vi "DataPacker_ConnectToMIDAS.vi"(8 "error in (no error)":errorcluster, 11 "DataPacker in":refnum<class "DataPacker.lvclass">) -> (0 "error out":errorcluster, 2 "MIDAS Reply":string, 3 "DataPacker out":refnum<class "DataPacker.lvclass">)   [LabVIEW 2018, in "feGEM DataPacker.lvlib" / "DataPacker.lvclass"]
uses:
  DataPacker.lvclass
  DataPacker.lvclass/DataPacker.ctl
  DataStructures/GEM_BANK_ARRAY.lvclass
  DataStructures/GEM_BANK_CLUSTER_typedef.ctl
  DataStructures/GEM_DATA_cluster_typedef.ctl
  5450c936-4932-4056-bb20-e5a86d0e2a98.vi
  feGEM DataPacker.lvlib
panel:
  out "Hostname of this PC":string
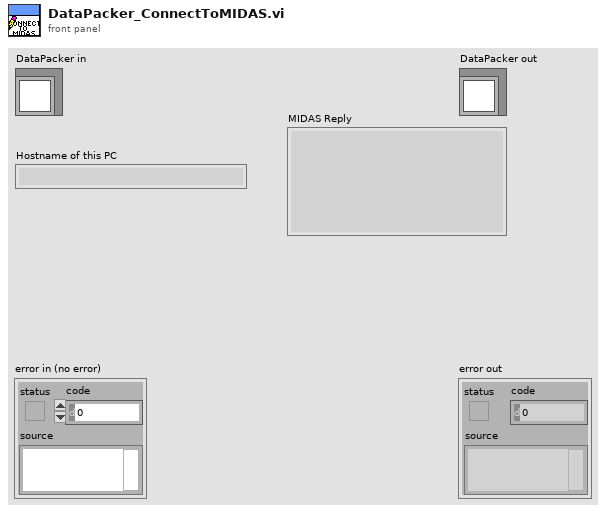
[diagram p1: front panel]
types:
  T1 = typedef "feGEM DataPacker.lvlib/GEM_BANK_CLUSTER_typedef.ctl" = cluster{"Category":string, "Variable Name":string, "Equipment description":string, "History Settings":u16, "Period to update history plots":u16, "GEM_DATA Cluster":T2}
  T2 = typedef "feGEM DataPacker.lvlib/GEM_DATA_cluster_typedef.ctl" = cluster{"DataType":string, "Formatted Data":u8[], "data byte order (Little Endian prefered)":enum16{"big-endian, network order", "native, host order", "little-endian"}}
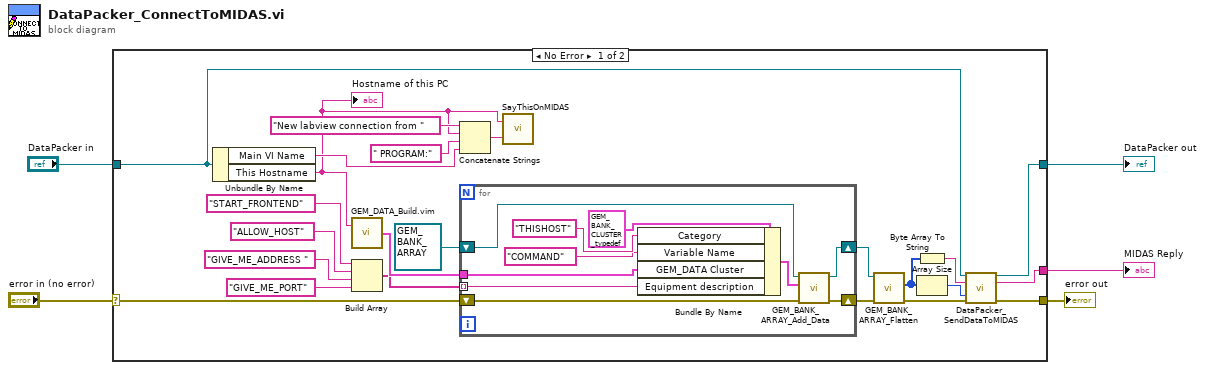
[diagram p0: block diagram]
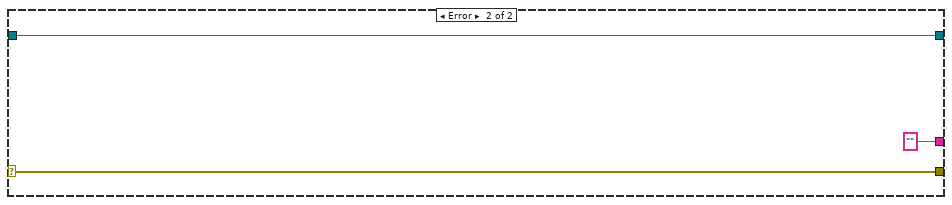
[diagram p2: hidden frame]
diagram:
  n1 = case shown="No Error" "error in (no error)" {
    selector: "error in (no error)" -> [w20 w40]
    tunnel: [w16 w40] -> w4
    tunnel: [w19 w41] -> w2
    tunnel: "DataPacker in" -> [w12 w41]
    tunnel: [w11 "" ("MIDAS Reply")] -> w1
    frame No Error {
      n2 = Unbundle By Name(w12) -> ("Main VI Name"=w10:string, "This Hostname"=w6:string)
      "Hostname of this PC" <- w6
      n3 = call "GEM_DATA_Build.vim"("Any array in"=w6) -> ("GEM_BANK Cluster"=w22:T2)  [unwired: 1 in]
      n4 = Build Array("START_FRONTEND" ("Variable Name"), "ALLOW_HOST" ("Variable Name"), "GIVE_ME_ADDRESS " ("data"), "GIVE_ME_PORT" ("Var Name")) -> (w7:string[])
      n5 = Concatenate Strings("New labview connection from ", w6, " PROGRAM:" ("string"), w10) -> (w13:string)
      n6 = for {
        tunnel: w22 -> [w31]
        shift-right: [w38] -> w27
        shift-left: refnum<class "GEM_BANK_ARRAY.lvclass"> refnum ("LVBANKARRAY.lvclass") -> [w37]
        shift-right: [w36] -> w26
        shift-left: w20 -> [w35]
        tunnel: w7 -> [w30] mode=indexing
        n7 = Bundle By Name(cluster=T1 {"Category"="", "Variable Name"="", "Equipment description"="", "History Settings"=0, "Period to update history plots"=0, "GEM_DATA Cluster"={"DataType"="", "Formatted Data"=[], "data byte order (Little Endian prefered)"=enum."big-endian, network order"}} ("output cluster"), "Category"="THISHOST", "Variable Name"="COMMAND", "GEM_DATA Cluster"=w31, "Equipment description"=w30) -> (w33:T1)
        n8 = call "GEM_BANK_ARRAY_Add_Data.vi"("error in (no error)"=w35, "GEM BANK Cluster"=w33, "LVBANKARRAY in"=w37) -> ("error out"=w36:errorcluster, "LVBANKARRAY out"=w38:refnum<class "GEM_BANK_ARRAY.lvclass">)  [unwired: 7 in]
      }
      n9 = call "SayThisOnMIDAS.vi"("String"=w13, "Hostname (Optional)"=w6) -> ()  [unwired: 1 out]
      n10 = call "GEM_BANK_ARRAY_Flatten.vi"("error in (no error)"=w26, "LVBANKARRAY in"=w27) -> ("error out"=w17:errorcluster, "Array"=w9:u8[])  [unwired: 7 in, 1 out]
      n11 = Byte Array To String(unsigned byte array=w9) -> (string=w18:string)
      n12 = Array Size(array=w9) -> (size(s)=w8:i32)
      n13 = call "DataPacker_SendDataToMIDAS.vi"("DataPacker in"=w12, "data in"=w18, "data in length"=w8, "error in (no error)"=w17) -> ("DataPacker out"=w19:refnum<class "DataPacker.lvclass">, "MIDAS Reply"=w11:string, "error out"=w16:errorcluster)  [unwired: 7 in, 2 out]
    }
    frame Error {
    }
  }
  "error out" <- w4
  "DataPacker out" <- w2
  "MIDAS Reply" <- w1
